vi "Write Image.vi"(0 "image in":refnum<class "MSC Image.lvclass">, 1 "image path":path, 2 "PNG Compression":i32, 3 "JPEG Quality":i32=100, 5 "error in (no error)":errorcluster, 8 "write image properties":bool, 10 "image properties path":path) -> (14 "image out":refnum<class "MSC Image.lvclass">, 19 "error out":errorcluster)   [LabVIEW 2016, in "MSC Image.lvclass"]
doc: "Saves the image to HD with optional PNG compression and JPEG quality setting. If \"write image properties\" is set to TRUE, a .ini file is created with image properties and variant data.\n\nSupported formats:\nWindows bitmaps, JPEG, JPEG 2000, Portable Network Graphics, Portable image format, Sun rasters, TIFF"
uses:
  MSC Image.lvclass
  Dependencies/x86/MSC I Process32.dll
  <vilib>/Utility/config.llb/NI_LVConfig.lvlib
  controls/Image Type.ctl
  controls/Size.ctl
  controls/INI Image Properties.vi
  <userlib>/_OpenG.lib/file/file.llb/Strip Path Extension - Path__ogtk.vi
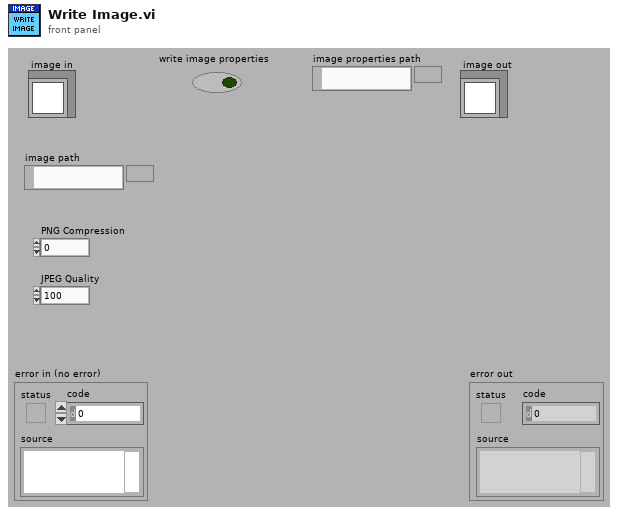
[diagram p1: front panel]
types:
  T1 = typedef "MSC Image.lvclass/INI Image Properties.vi" = cluster{"Size":T2, "Image Type":T3, "Timestamp":string, "Variant":variant}
  T2 = typedef "MSC Image.lvclass/Size.ctl" = cluster{"Cols":i32, "Rows":i32}
  T3 = typedef "MSC Image.lvclass/Image Type.ctl" = i32
  T4 = enum16{"open", "replace", "create", "open or create", "replace or create", "replace or create with confirmation"}
  T5 = typedef "Image.ctl" = cluster{"Pointer":u64, "Size":T6, "Image Type":T7, "Time Stamp":timestamp, "Variant":variant}
  T6 = typedef "Size.ctl" = cluster{"Cols":i32, "Rows":i32}
  T7 = typedef "Image Type.ctl" = i32
  T8 = typedef "MSC Image.lvclass/Image.ctl" = cluster{"Pointer":u64, "Size":T2, "Image Type":T3, "Time Stamp":timestamp, "Variant":variant}
  T9 = typedef "NI_LVConfig.lvlib/Config Data RefNum.ctl" = refnum<k1>
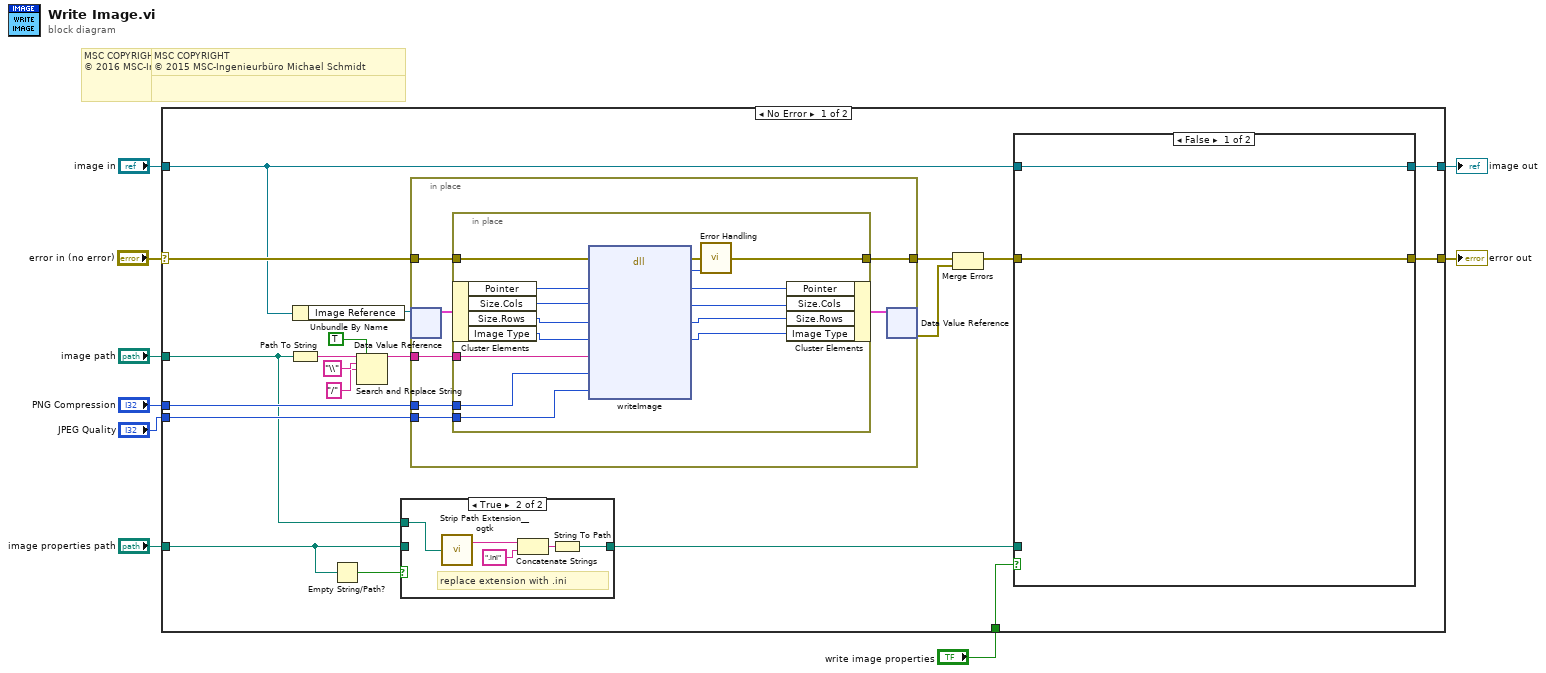
[diagram p0: block diagram]
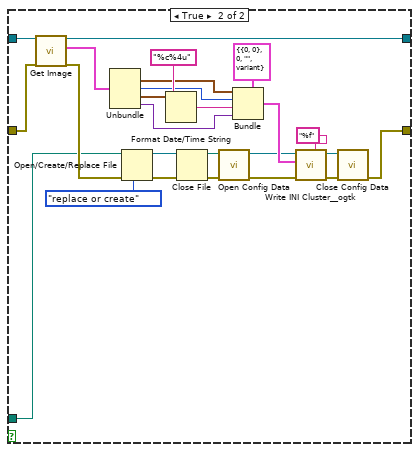
[diagram p3: hidden frame]
diagram:
  # "MSC COPYRIGHT\n© 2016 MSC-Ingenieurbüro Michael Schmidt"
  # "MSC COPYRIGHT\n© 2016 MSC-Ingenieurbüro Michael Schmidt"
  # "MSC COPYRIGHT\n© 2015 MSC-Ingenieurbüro Michael Schmidt"
  # "MSC COPYRIGHT\n© 2015 MSC-Ingenieurbüro Michael Schmidt"
  n1 = case shown="No Error" "error in (no error)" {
    selector: "error in (no error)" -> [w26 w86]
    tunnel: [w15 w86] -> w5
    tunnel: [w17 w85] -> w9
    tunnel: "image in" -> [w18 w85]
    tunnel: "image path" -> [w11 _]
    tunnel: "PNG Compression" -> [w20 _]
    tunnel: "JPEG Quality" -> [w19 _]
    tunnel: "write image properties" -> [w14 _]
    tunnel: "image properties path" -> [w12 _]
    frame No Error {
      n2 = Path To String(path=w11) -> (string=w22:string)
      n3 = Unbundle By Name(w18) -> ("Image Reference"=w29:refnum<data-value>)
      n4 = Empty String/Path?(string/path=w12) -> (empty?=w13:bool)
      n5 = Search and Replace String(replace all?=TRUE ("replace all? (F)"), input string=w22, search string="\\", replace string="/" ("replace string (\"\")")) -> (result string=w21:string)  [unwired: 4 in, 3 out]
      n6 = case shown="True" w13 {
        tunnel: w12 -> [w30 _]
        tunnel: [w30 w31] -> w10
        tunnel: w11 -> [_ w35]
        frame False {
        }
        frame True {
          # "replace extension with .ini"
          n7 = call-poly <userlib>:"Strip Path Extension__ogtk.vi"("path"=w35) -> ("root"=w34:string)  [unwired: 1 out]
          n8 = Concatenate Strings(w34, ".ini" ("string")) -> (w32:string)
          n9 = String To Path(string=w32) -> (path=w31:path)
        }
      }
      n10 = in-place {
        in-place-border: w26 -> [w67]
        in-place-border: [w66] -> w28
        in-place-border: w21 -> [w65]
        in-place-border: w20 -> [w64]
        in-place-border: w19 -> [w63]
        n11 = in-place-dvr #1(w29) -> (w68:T5)  [unwired: 1 out]
        n12 = in-place {
          in-place-border: w67 -> [w72]
          in-place-border: [w79] -> w66
          in-place-border: w65 -> [w73]
          in-place-border: w64 -> [w71]
          in-place-border: w63 -> [w70]
          n13 = in-place-cluster #2(w68) -> ("Pointer"=w82:u64, "Size.Cols"=w83:i32, "Size.Rows"=w84:i32, "Image Type"=w76:T7)
          n14 = dll-call lib="C:/Users/MSC/LabVIEW Projekte/LV 2014/MSC I-Process/user.lib/MSC-I Process/Dependencies/x86/MSC I Process*.dll" fn="writeImage"(error in=w72, "pointer"=w82, "cols"=w83, "rows"=w84, "type"=w76, "pathString"=w73, "pngCompression"=w71, "jpegQuality"=w70) -> (error out=w80:errorcluster, "error"=w81:i32, "pointer"=w74:u64, "cols"=w78:i32, "rows"=w77:i32, "type"=w75:i32)  [unwired: 5 in, 1 out]
          n15 = call "Error Handling.vi"("error in (no error)"=w80, "return type"=w81) -> ("error out"=w79:errorcluster)  [unwired: 12 in, 1 out]
          n16 = in-place-cluster #2("Pointer"=w74, "Size.Cols"=w78, "Size.Rows"=w77, "Image Type"=w75) -> (w69:T5)
        }
        n17 = in-place-dvr #1(w69) -> (w27:errorcluster)  [unwired: 1 out]
      }
      n18 = Merge Errors(w28, w27) -> (w16:errorcluster)
      n19 = case shown="False" w14 {
        tunnel: w18 -> [w37 w62]
        tunnel: [w37 w61] -> w17
        tunnel: w16 -> [w36 w60]
        tunnel: [w36 w40] -> w15
        tunnel: w10 -> [_ w38]
        frame False {
        }
        frame True {
          n20 = call-dynamic "Get Image.vi"("image in"=w62, "error in (no error)"=w60) -> ("image out"=w61:refnum<class "MSC Image.lvclass">, "Image"=w45:T8, "error out"=w39:errorcluster)  [unwired: 15 in]
          n21 = Unbundle(w45) -> ("Size"=w44:T2, "Image Type"=w43:T3, "Time Stamp"=w42:timestamp, "Variant"=w41:variant)  [unwired: 1 out]
          n22 = Open/Create/Replace File(file path (use dialog)=w38, error in=w39, operation (0:open)=T4."replace or create") -> (refnum out=w52:refnum<file>, error out=w51:errorcluster)  [unwired: 3 in, 1 out]
          n23 = Format Date/Time String(time format string (%c)="%c%4u", seconds (now)=w42) -> (date/time string=w57:string)  [unwired: 1 in]
          n24 = Close File(refnum=w52, error in=w51) -> (path=w53:path, error out=w58:errorcluster)
          n25 = call <vilib>:"Open Config Data.vi"("error in (no error)"=w58, "configuration file path"=w53) -> ("error out"=w46:errorcluster, "refnum"=w47:T9)  [unwired: 7 in, 1 out]
          n26 = Bundle(cluster=T1 {"Size"={"Cols"=0, "Rows"=0}, "Image Type"=0, "Timestamp"="", "Variant"=variant} ("CSV Image Properties"), "Size"=w44, "Image Type"=w43, "Timestamp"=w57, "Variant"=w41) -> (w55:T1)
          n27 = call <userlib>:"Write INI Cluster__ogtk.vi"("float number format (optional)"="%f", "error in (no error)"=w46, "INI Fomatted Cluster"=w55, "refnum"=w47) -> ("error out"=w48:errorcluster, "dup refnum"=w49:T9)  [unwired: 6 in]
          n28 = call <vilib>:"Close Config Data.vi"("error in (no error)"=w48, "refnum"=w49) -> ("error out"=w40:errorcluster)  [unwired: 8 in, 1 out]
        }
      }
    }
    frame Error {
    }
  }
  "error out" <- w5
  "image out" <- w9
